vi "Dummy.vi"(8 "error in (no error)":errorcluster, 10 "Numeric":dbl, 11 "Test Interface in":refnum<class "Test Interface Pure Mock.lvclass">) -> (0 "error out":errorcluster, 2 "Boolean":bool, 3 "Test Interface out":refnum<class "Test Interface Pure Mock.lvclass">)   [LabVIEW 2020, in "Test Interface Pure Mock.lvclass"]
uses:
  Test Interface Pure Mock.lvclass
  C:/Program Files (x86)/National Instruments/LabVIEW 2020/vi.lib/Astemes/LMock/Pure Mock.lvclass
  Test Interface Pure Mock.lvclass/Test Interface Pure Mock.ctl
  <vilib>/Astemes/LMock/Pure Mock.lvclass
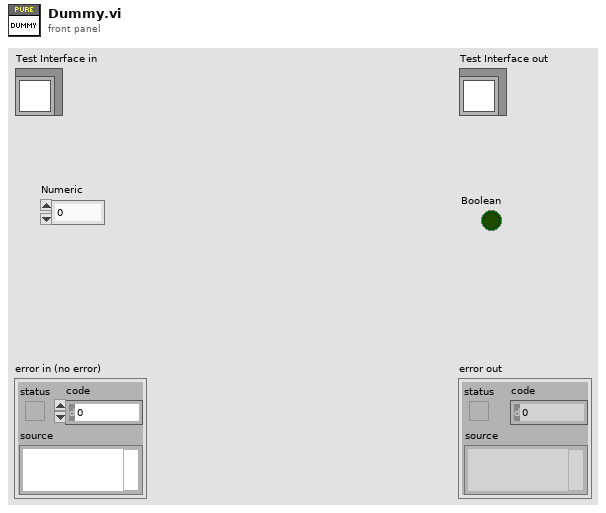
[diagram p1: front panel]
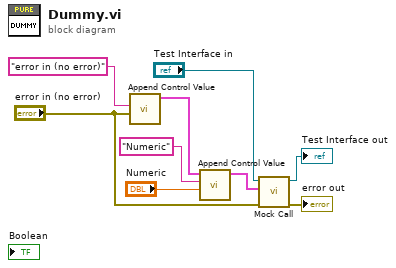
[diagram p0: block diagram]
diagram:
  n1 = call <vilib>:"Append Control Value.vi"("Variant Data"="error in (no error)", "Name"="error in (no error)") -> ("Array"=w2:cluster{"Name":string, "Variant Data":variant}[])  [unwired: 9 in]
  n2 = call <vilib>:"Append Control Value.vi"("Variant Data"="Numeric", "Name"="Numeric", "Control Values"=w2) -> ("Array"=w5:cluster{"Name":string, "Variant Data":variant}[])  [unwired: 8 in]
  n3 = call <vilib>:"Mock Call.vi"("error in (no error)"="error in (no error)", "Control Values"=w5, "Mock In"="Test Interface in") -> ("error out"=→"error out":errorcluster, "Mock Out"=→"Test Interface out":refnum<class "Test Interface Pure Mock.lvclass">)  [unwired: 7 in]
